vi "Task Start.vi"(8 "error in (no error)":errorcluster, 11 "SimTask in":refnum<class "SimTask.lvclass">) -> (0 "error out":errorcluster, 3 "SimTask out":refnum<class "SimTask.lvclass">)   [LabVIEW 2020, in "VolatusDemo.lvlib" / "SimTask.lvclass"]
uses:
  SimTask.lvclass
  SimTask.lvclass/SimTask.ctl
  Volatus/Task/Task.lvclass
  VolatusData/DataProcessor/DataProcessor.lvclass
  VolatusConfig/Task/Task.lvclass
  VolatusConfig/VolatusConfigElement/VolatusConfigElement.lvclass
  C:/dev/lv20CE/relink/lv-volatus/Volatus/Task/Task.lvclass
  C:/Program Files (x86)/National Instruments/LabVIEW 2020/vi.lib/ActorFramework/Actor/Actor.lvclass
  C:/dev/lv20CE/relink/lv-volatus/Volatus/TaskStateHandler/TaskStateHandler.lvclass
  C:/dev/lv20CE/relink/lv-volatus/Volatus/VectoMessageHandler/VectoMessageHandler.lvclass
  C:/dev/lv20CE/relink/lv-volatus/VolatusDemo/SimTask/SimTask.lvclass
  C:/dev/lv20CE/relink/lv-volatus/VolatusConfig/VolatusConfigElement/VolatusConfigElement.lvclass
  C:/dev/lv20CE/relink/lv-volatus/VolatusConfig/Task/Task.lvclass
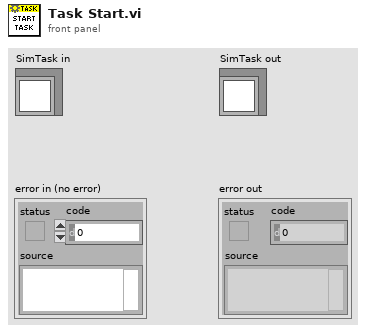
[diagram p1: front panel]
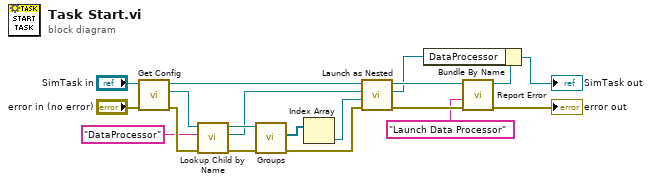
[diagram p0: block diagram]
diagram:
  n1 = call "Get Config.vi"("error in (no error)"="error in (no error)", "Task in"="SimTask in") -> ("error out"=w9:errorcluster, "Config"=w4:refnum<class "Task.lvclass">, "Task out"=w10:refnum<class "SimTask.lvclass">)  [unwired: 7 in]
  n2 = call "Lookup Child by Name.vi"("error in (no error)"=w9, "Child Name"="DataProcessor", "VolatusConfigElement in"=w4) -> ("error out"=w5:errorcluster, "Child"=w1:refnum<class "Config Element.lvclass">, "VolatusConfigElement out"=w3:refnum<class "Task.lvclass">)  [unwired: 5 in, 1 out]
  n3 = call "Groups.vi"("error in (no error)"=w5, "Task in"=w3) -> ("error out"=w7:errorcluster, "Groups"=w8:refnum<class "Group.lvclass">[])  [unwired: 7 in, 1 out]
  n4 = Index Array(array=w8) -> (element=w6:refnum<class "Group.lvclass">)  [unwired: 1 in]
  n5 = call "Launch as Nested.vi"("error in (no error)"=w7, "Group Config"=w6, "DataProcessor Config"=w1, "Parent Task in"=w10) -> ("error out"=w19:errorcluster, "API"=w12:refnum<class "DataHandlerAPI.lvclass">, "Parent Task"=w13:refnum<class "SimTask.lvclass">)  [unwired: 5 in]
  n6 = call "Report Error.vi"("error in (no error)"=w19, "Message"="Launch Data Processor", "Task in"=w13) -> ("error out"=→"error out":errorcluster, "Task out"=w16:refnum<class "SimTask.lvclass">)  [unwired: 7 in]
  n7 = Bundle By Name(cluster=w16, "DataProcessor"=w12) -> (→"SimTask out":refnum<class "SimTask.lvclass">)
